vi "ROB info data insert.vi"(8 "error in (no error)":errorcluster, 10 "Data in":u8[](array[numeric]), 11 "Hist cluster":refnum<vi>) -> (0 "error out":errorcluster)   [LabVIEW 2016]
uses:
  <vilib>/Utility/miscctls.llb/LVRowAndColumnTypeDef.ctl
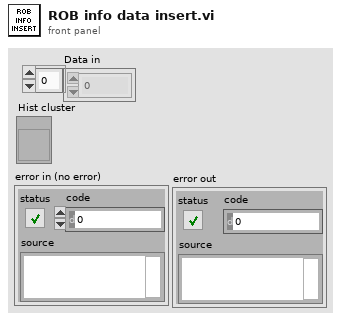
[diagram p1: front panel]
types:
  T1 = typedef "ROB info refnum.ctl" = refnum<vi>
  T2 = typedef "ROB display info.ctl" = cluster{"ID:":i32, "State:":string, "Voltages":i32, "Temp:":dbl, "Latch count:":i32, "VRef:":enum16{"External", "Internal", "Unknown"}, "Trigthres:":i32, "MPPC EN":bool, "Test charge":bool, "Responding":bool, "Last update":timestamp}
  T3 = typedef "All ROBs info cluster refnum.ctl" = refnum<vi>
  T4 = cluster{"Long":i32, "Float":dbl, "Bool":bool, "Byte":u8, "Byte array":u8[]}
  T5 = enum16{"Byte array", "Byte", "Bool", "Long", "Float"}
  T6 = enum16{"ID", "Status", "Voltages", "Temp", "Latch count", "VRef", "Trigthres", "MPPC EN?", "Test charge?", "Responding?"}
  T7 = typedef "LVRowAndColumnTypeDef.ctl" = cluster{"Row":i32, "Column":i32}
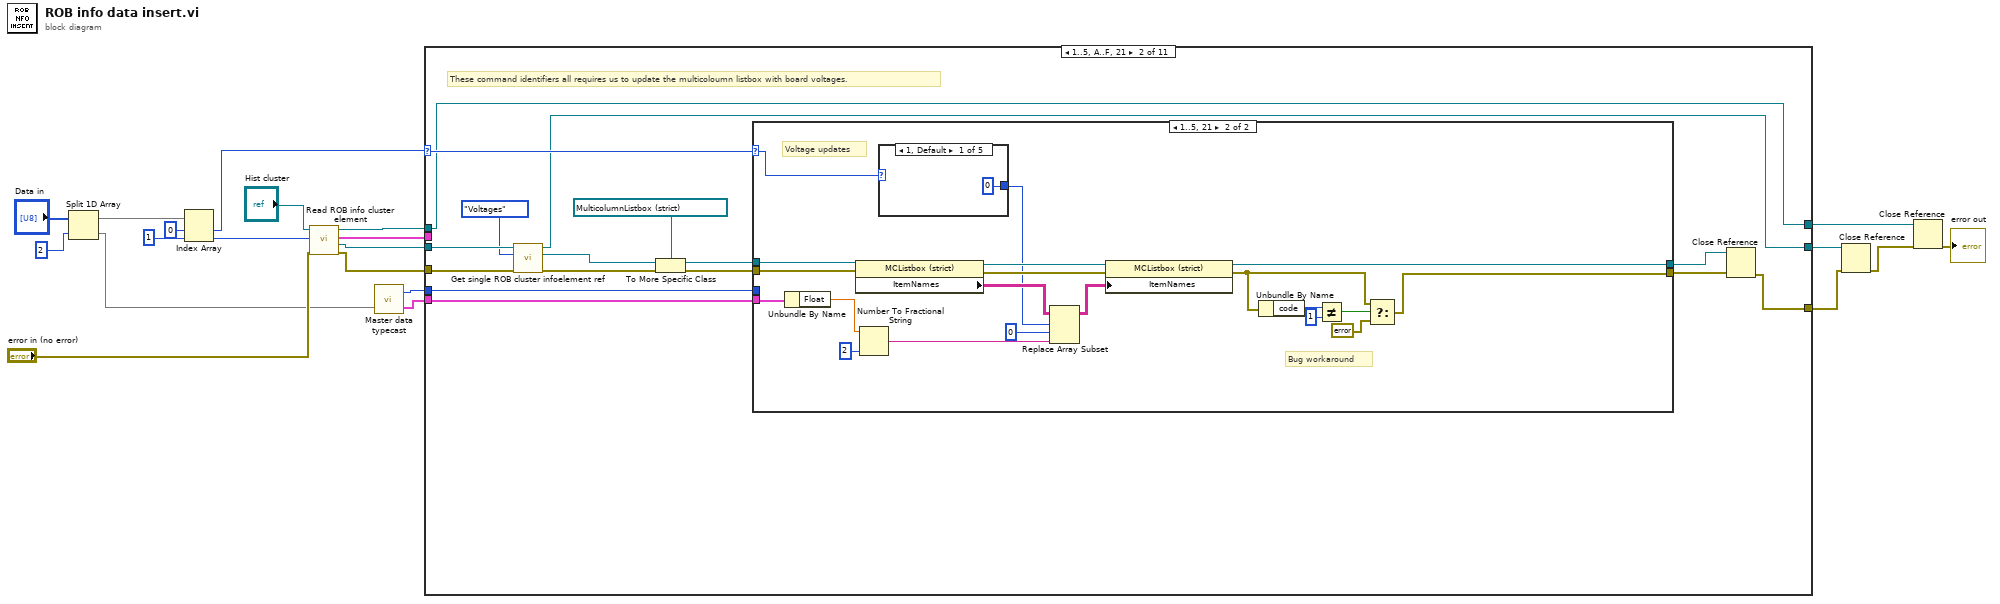
[diagram p0: block diagram]
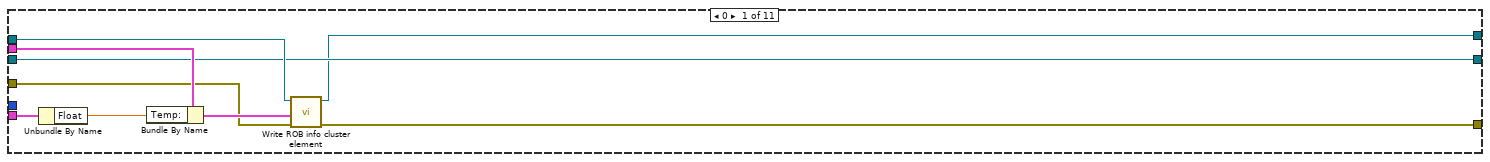
[diagram p2: hidden frame]
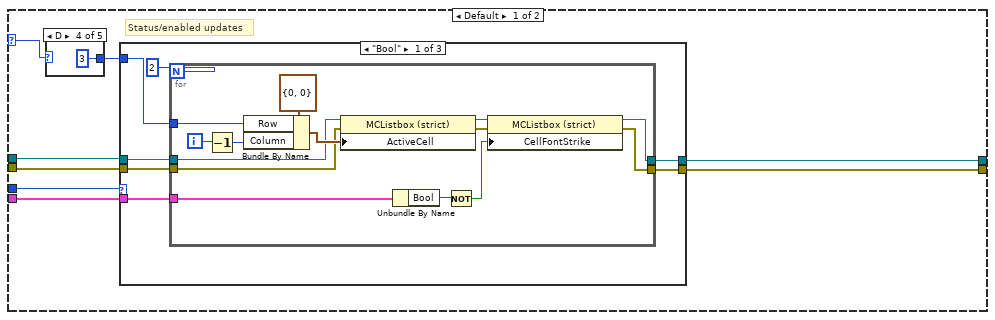
[diagram p3: hidden frame]
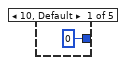
[diagram p4: hidden frame]
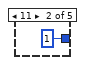
[diagram p5: hidden frame]
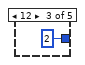
[diagram p6: hidden frame]
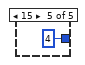
[diagram p7: hidden frame]
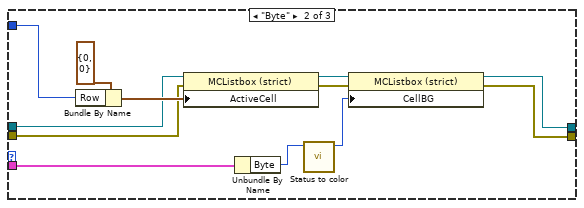
[diagram p8: hidden frame]
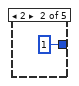
[diagram p10: hidden frame]
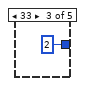
[diagram p11: hidden frame]
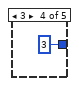
[diagram p12: hidden frame]
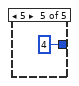
[diagram p13: hidden frame]
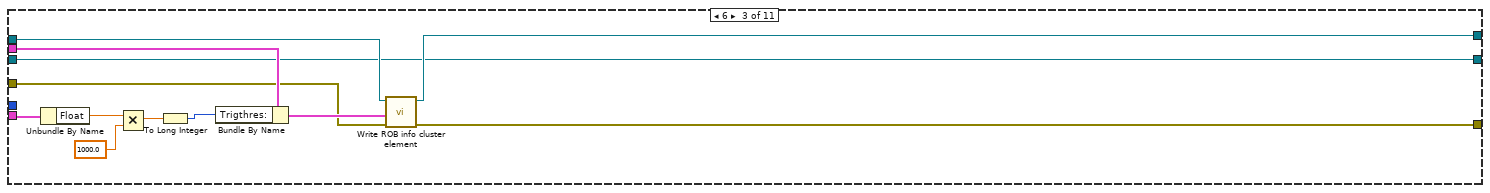
[diagram p14: hidden frame]
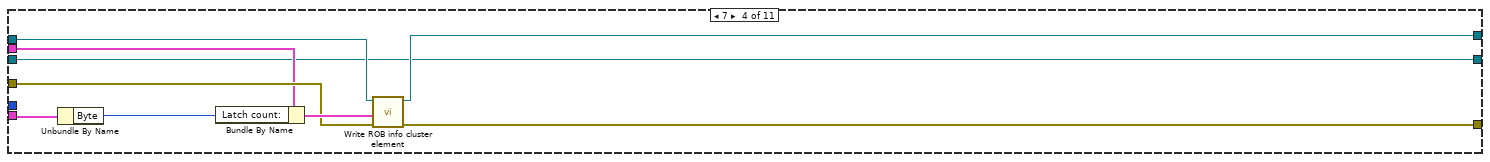
[diagram p15: hidden frame]
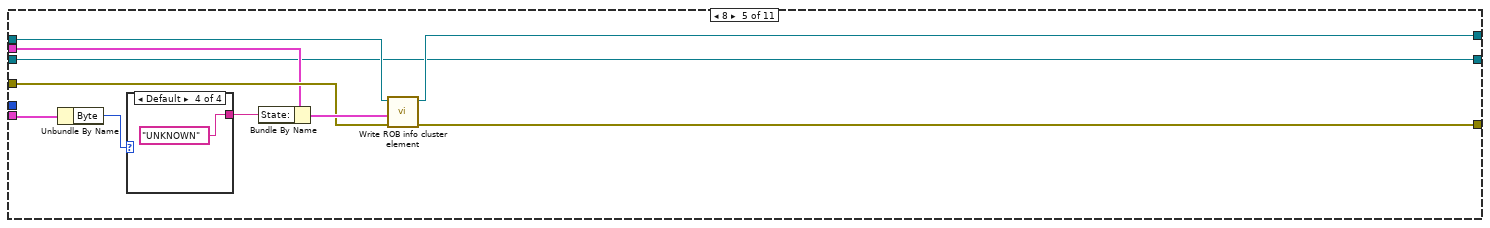
[diagram p16: hidden frame]
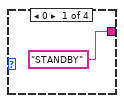
[diagram p17: hidden frame]
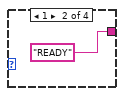
[diagram p18: hidden frame]
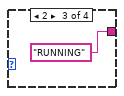
[diagram p19: hidden frame]
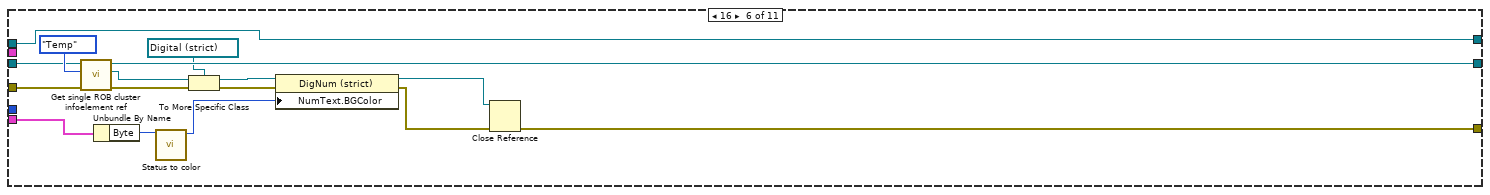
[diagram p20: hidden frame]
diagram:
  n1 = Split 1D Array(array="Data in", index=2) -> (first subarray=w13:u8[], second subarray=w12:u8[])
  n2 = Index Array(array=w13, index #1=0 ("index"), index #2=1 ("index")) -> (element #1=w17:u8, element #2=w20:u8)
  n3 = call "Read ROB info cluster element.vi"("error in (no error)"="error in (no error)", "Channel"=w20, "ROB info clusters"="Hist cluster") -> ("error out"=w9:errorcluster, "ROB infocluster ref"=w10:T1, "ROB Info-display"=w16:T2, "ROB info clusters"=w7:T3)  [unwired: 5 in]
  n4 = call "Master data typecast.vi"("Data in"=w12) -> ("Data out"=w11:T4, "Datatype"=w8:T5)  [unwired: 1 in]
  n5 = case shown="1..5, A..F, 21" w17 {
    selector: w17 -> [_ w39 _ _ _ _ _ _ _ _ _]
    tunnel: w16 -> [w30 _ w130 w137 w148 _ _ w195 w204 w214 _]
    tunnel: w11 -> [w29 w46 w128 w135 w146 w163 w179 w194 w203 w213 _]
    tunnel: w10 -> [w24 w45 w125 w133 w144 w168 w184 w188 w197 w208 w220]
    tunnel: w9 -> [w25 w44 w124 w138 w149 w169 w185 w191 w200 w211 w218]
    tunnel: w8 -> [_ w38 _ _ _ _ _ _ _ _ _]
    tunnel: w7 -> [w26 w34 w129 w136 w147 w159 w175 w190 w199 w210 w219]
    tunnel: [w24 w32 w125 w133 w144 w160 w176 w188 w197 w208 w220] -> w6
    tunnel: [w23 w34 w126 w134 w145 w159 w175 w189 w198 w209 w219] -> w5
    tunnel: [w22 w35 w127 w132 w141 w156 w172 w187 w196 w205 w218] -> w3
    frame 0 {
      n6 = Unbundle By Name(w29) -> ("Float"=w28:dbl)
      n7 = Bundle By Name(cluster=w30, "Temp:"=w28) -> (w27:T2)
      n8 = call "Write ROB info cluster element.vi"("error in (no error)"=w25, "ROB Info-display"=w27, "Hist cluster"=w26) -> ("error out"=w22:errorcluster, "Hist cluster"=w23:T3)  [unwired: 7 in]
    }
    frame 1..5, 10..15, 33 {
      # "These command identifiers all requires us to update the multicoloumn listbox with board voltages."
      n9 = call "Get single ROB cluster infoelement ref.vi"("error in (no error)"=w44, "Enum"=T6."Voltages", "ROB infocluster ref"=w45) -> ("error out"=w43:errorcluster, "Element reference"=w33:refnum<vi>, "ROB infocluster ref"=w32:T1)  [unwired: 6 in]
      n10 = To More Specific Class(target class=refnum<vi> refnum ("Voltages"), reference=w33, error in=w43) -> (specific class reference=w41:refnum<vi>, error out=w40:errorcluster)
      n11 = case shown="1..5, 21" w39 {
        selector: w39 -> [w53 w104]
        tunnel: w46 -> [w52 w114]
        tunnel: w41 -> [w48 w113]
        tunnel: w40 -> [w47 w112]
        tunnel: [w50 w101] -> w36
        tunnel: [w51 w96] -> w37
        tunnel: w38 -> [w54 _]
        frame Default {
          # "Status/enabled updates"
          n12 = case shown="D" w53 {
            tunnel: [0 ("index (row)") 1 ("index (row)") 2 ("index (row)") 3 ("index (row)") 4 ("index (row)")] -> w49
            frame 10, Default {
            }
            frame 11 {
            }
            frame 12 {
            }
            frame 13 {
            }
            frame 15 {
            }
          }
          n13 = case shown="\"Bool\"" w54 {
            tunnel: w47 -> [w62 w82 w93]
            tunnel: w48 -> [w61 w81 w94]
            tunnel: w52 -> [w66 w92 _]
            tunnel: [w65 w89 w93] -> w51
            tunnel: [w64 w88 w94] -> w50
            tunnel: w49 -> [w63 w83 _]
            frame "Bool" {
              n14 = for {
                N: 2 -> [_]
                tunnel: w66 -> [w80]
                tunnel: [w77] -> w65
                tunnel: [w76] -> w64
                tunnel: w63 -> [w73]
                tunnel: w62 -> [w70]
                tunnel: w61 -> [w69]
                i -> [w68]
                n15 = Decrement(x=w68) -> (x-1=w67:i32)
                n16 = Bundle By Name(cluster=T7 {"Row"=0, "Column"=0} ("Active Cell:Active Cell"), "Row"=w73, "Column"=w67) -> (w74:T7)
                n17 = property class="MCListbox (strict)"(reference=w69, error in=w70, "ActiveCell"=w74) -> (reference out=w71:refnum<vi>, error out=w72:errorcluster)
                n18 = Unbundle By Name(w80) -> ("Bool"=w79:bool)
                n19 = Not(x=w79) -> (.not. x?=w78:bool)
                n20 = property class="MCListbox (strict)"(reference=w71, error in=w72, "CellFontStrike"=w78) -> (reference out=w76:refnum<vi>, error out=w77:errorcluster)
              }
            }
            frame "Byte" {
              n21 = Bundle By Name(cluster=T7 {"Row"=0, "Column"=0} ("Active Cell:Active Cell"), "Row"=w83) -> (w86:T7)
              n22 = property class="MCListbox (strict)"(reference=w81, error in=w82, "ActiveCell"=w86) -> (reference out=w85:refnum<vi>, error out=w84:errorcluster)
              n23 = Unbundle By Name(w92) -> ("Byte"=w91:u8)
              n24 = call "Status to color.vi"("Byte"=w91) -> ("Numeric"=w90:u32)  [unwired: 10 in]
              n25 = property class="MCListbox (strict)"(reference=w85, error in=w84, "CellBG"=w90) -> (reference out=w88:refnum<vi>, error out=w89:errorcluster)
            }
            frame Default {
            }
          }
        }
        frame 1..5, 33 {
          # "Bug workaround"
          # "Voltage updates"
          n26 = Unbundle By Name(w114) -> ("Float"=w110:dbl)
          n27 = property class="MCListbox (strict)"(reference=w113, error in=w112) -> (reference out=w107:refnum<vi>, error out=w106:errorcluster, "ItemNames"=w111:string[][])
          n28 = Number To Fractional String(number=w110, precision (6)=i16 2) -> (F-format string=w108:string)  [unwired: 2 in]
          n29 = case shown="1, Default" w104 {
            tunnel: [0 ("index (row)") 1 ("index (row)") 2 ("index (row)") 3 ("index (row)") 4 ("index (row)")] -> w102
            frame 1, Default {
            }
            frame 2 {
            }
            frame 33 {
            }
            frame 3 {
            }
            frame 5 {
            }
          }
          n30 = Replace Array Subset(array=w111, new element=w108, index (row)=w102, index (col)=0 ("disabled index (col)")) -> (w105:string[][])
          n31 = property class="MCListbox (strict)"(reference=w107, error in=w106, "ItemNames"=w105) -> (reference out=w101:refnum<vi>, error out=w97:errorcluster)
          n32 = Unbundle By Name(w97) -> ("code"=w100:i32)
          n33 = Not Equal?(x=w100, y=1) -> (x != y?=w98:bool)
          n34 = Select(t=w97, s=w98, f=errorcluster {"status"=FALSE, "code"=0, "source"=""}) -> (s? t:f=w96:errorcluster)
        }
      }
      n35 = Close Reference(reference=w36, error in (no error)=w37) -> (error out=w35:errorcluster)
    }
    frame 6 {
      n36 = Unbundle By Name(w128) -> ("Float"=w123:dbl)
      n37 = Multiply(x=w123, y=1000.0) -> (x*y=w121:dbl)
      n38 = To Long Integer(number=w121) -> (32bit integer=w120:i32)
      n39 = Bundle By Name(cluster=w130, "Trigthres:"=w120) -> (w131:T2)
      n40 = call "Write ROB info cluster element.vi"("error in (no error)"=w124, "ROB Info-display"=w131, "Hist cluster"=w129) -> ("error out"=w127:errorcluster, "Hist cluster"=w126:T3)  [unwired: 7 in]
    }
    frame 7 {
      n41 = Unbundle By Name(w135) -> ("Byte"=w140:u8)
      n42 = Bundle By Name(cluster=w137, "Latch count:"=w140) -> (w139:T2)
      n43 = call "Write ROB info cluster element.vi"("error in (no error)"=w138, "ROB Info-display"=w139, "Hist cluster"=w136) -> ("error out"=w132:errorcluster, "Hist cluster"=w134:T3)  [unwired: 7 in]
    }
    frame 8 {
      n44 = Unbundle By Name(w146) -> ("Byte"=w143:u8)
      n45 = case shown="Default" w143 {
        tunnel: ["STANDBY" "READY" "RUNNING" "UNKNOWN"] -> w142
        frame 0 {
        }
        frame 1 {
        }
        frame 2 {
        }
        frame Default {
        }
      }
      n46 = Bundle By Name(cluster=w148, "State:"=w142) -> (w150:T2)
      n47 = call "Write ROB info cluster element.vi"("error in (no error)"=w149, "ROB Info-display"=w150, "Hist cluster"=w147) -> ("error out"=w141:errorcluster, "Hist cluster"=w145:T3)  [unwired: 7 in]
    }
    frame 16 {
      n48 = call "Get single ROB cluster infoelement ref.vi"("error in (no error)"=w169, "Enum"=T6."Temp", "ROB infocluster ref"=w168) -> ("error out"=w166:errorcluster, "Element reference"=w167:refnum<vi>, "ROB infocluster ref"=w160:T1)  [unwired: 6 in]
      n49 = Unbundle By Name(w163) -> ("Byte"=w162:u8)
      n50 = call "Status to color.vi"("Byte"=w162) -> ("Numeric"=w161:u32)  [unwired: 10 in]
      n51 = To More Specific Class(target class=refnum<vi> refnum ("Numeric"), reference=w167, error in=w166) -> (specific class reference=w165:refnum<vi>, error out=w164:errorcluster)
      n52 = property class="DigNum (strict)"(reference=w165, error in=w164, "NumText.BGColor"=w161) -> (reference out=w157:refnum<vi>, error out=w158:errorcluster)
      n53 = Close Reference(reference=w157, error in (no error)=w158) -> (error out=w156:errorcluster)
    }
    frame 17 {
      n54 = call "Get single ROB cluster infoelement ref.vi"("error in (no error)"=w185, "Enum"=T6."Latch count", "ROB infocluster ref"=w184) -> ("error out"=w182:errorcluster, "Element reference"=w183:refnum<vi>, "ROB infocluster ref"=w176:T1)  [unwired: 6 in]
      n55 = Unbundle By Name(w179) -> ("Byte"=w178:u8)
      n56 = call "Status to color.vi"("Byte"=w178) -> ("Numeric"=w177:u32)  [unwired: 10 in]
      n57 = To More Specific Class(target class=refnum<vi> refnum ("Latch count:"), reference=w183, error in=w182) -> (specific class reference=w181:refnum<vi>, error out=w180:errorcluster)
      n58 = property class="DigNum (strict)"(reference=w181, error in=w180, "NumText.BGColor"=w177) -> (reference out=w173:refnum<vi>, error out=w174:errorcluster)
      n59 = Close Reference(reference=w173, error in (no error)=w174) -> (error out=w172:errorcluster)
    }
    frame 18 {
      n60 = Unbundle By Name(w194) -> ("Bool"=w193:bool)
      n61 = Bundle By Name(cluster=w195, "MPPC EN"=w193) -> (w192:T2)
      n62 = call "Write ROB info cluster element.vi"("error in (no error)"=w191, "ROB Info-display"=w192, "Hist cluster"=w190) -> ("error out"=w187:errorcluster, "Hist cluster"=w189:T3)  [unwired: 7 in]
    }
    frame 19 {
      n63 = Unbundle By Name(w203) -> ("Bool"=w202:bool)
      n64 = Bundle By Name(cluster=w204, "Test charge"=w202) -> (w201:T2)
      n65 = call "Write ROB info cluster element.vi"("error in (no error)"=w200, "ROB Info-display"=w201, "Hist cluster"=w199) -> ("error out"=w196:errorcluster, "Hist cluster"=w198:T3)  [unwired: 7 in]
    }
    frame 20 {
      n66 = Unbundle By Name(w213) -> ("Byte"=w207:u8)
      n67 = case shown="Default" w207 {
        tunnel: [enum16{"External", "Internal", "Unknown"}."Internal" ("VRef:") enum16{"External", "Internal", "Unknown"}."External" ("VRef:") enum16{"External", "Internal", "Unknown"}."Unknown" ("VRef:")] -> w206
        frame 0 {
        }
        frame 1 {
        }
        frame Default {
        }
      }
      n68 = Bundle By Name(cluster=w214, "VRef:"=w206) -> (w212:T2)
      n69 = call "Write ROB info cluster element.vi"("error in (no error)"=w211, "ROB Info-display"=w212, "Hist cluster"=w210) -> ("error out"=w205:errorcluster, "Hist cluster"=w209:T3)  [unwired: 7 in]
    }
    frame Default {
    }
  }
  n70 = Close Reference(reference=w6, error in (no error)=w3) -> (error out=w4:errorcluster)
  n71 = Close Reference(reference=w5, error in (no error)=w4) -> (error out=→"error out":errorcluster)
